vi "Set member data - outputs on.vi"(8 "error in (no error)":errorcluster, 10 "Array of outputs on?":bool[](array[boolean]), 11 "Function Generator.lvclass in":refnum<class "Function Generator.lvclass">) -> (0 "error out":errorcluster, 3 "Function Generator.lvclass out":refnum<class "Function Generator.lvclass">)   [LabVIEW 2015, in "Function Generator.lvclass"]
uses:
  Function Generator.lvclass
  Function Generator.lvclass/Function Generator.ctl
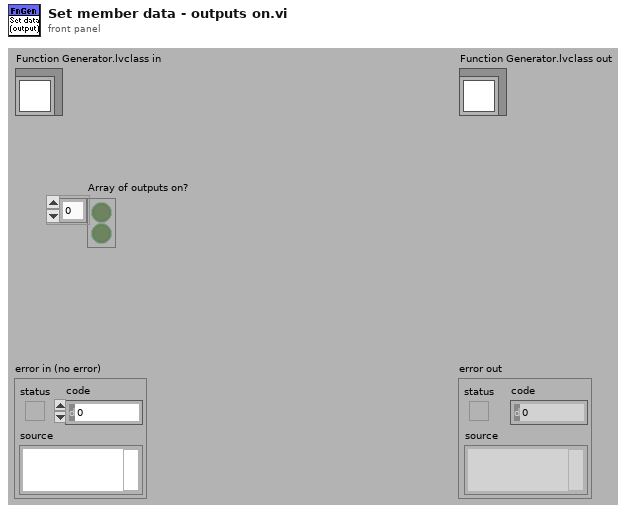
[diagram p1: front panel]
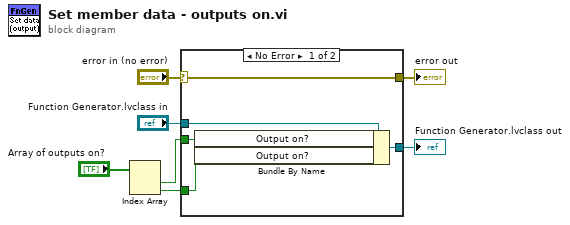
[diagram p0: block diagram]
diagram:
  n1 = Index Array(array="Array of outputs on?") -> (element #1=w2:bool, element #2=w1:bool)  [unwired: 2 in]
  n2 = case shown="No Error" "error in (no error)" {
    selector: "error in (no error)" -> [w12 w13]
    tunnel: [w12 w13] -> w6
    tunnel: [w10 w14] -> w4
    tunnel: "Function Generator.lvclass in" -> [w11 w14]
    tunnel: w2 -> [w9 _]
    tunnel: w1 -> [w8 _]
    frame No Error {
      n3 = Bundle By Name(cluster=w11, "Output on?"=w9, "Output on?"=w8) -> (w10:refnum<class "Function Generator.lvclass">)
    }
    frame Error {
    }
  }
  "error out" <- w6
  "Function Generator.lvclass out" <- w4
